vi "Initialize SRQ.vi"(8 "error in":errorcluster {"code" format="%.0x"}, 11 "dup VISA session":refnum<visa-resource-name>) -> (0 "error out (no error)":errorcluster {"code" format="%.0x"}, 3 "dup VISA session":refnum<visa-resource-name>)   [LabVIEW 2011]
doc: "Initializes VISA for a service request, discards any events already in the queue, then enables VISA event handling for a service request.\n\nThis VI is part of an SRQ operation sequence, the order of which is as follows:\n\n1) Set up instrument event-enable registers\n2) Call Initialize SRQ.vi\n3) Perform an operation that causes the instrument to generate a service request\n4) Call Wait on SRQ.vi\n\nor\n\n1) Set up instrument event enable registers\n2) Call Initialize SRQ.vi\n3) Perform the following in parallel using parallel loops or other LV event handling feature:\n - Perform operations that might cause the instrument to generate a service request\n - Call Check on SRQ.vi\n4) Handle any service request received\n5) Call Close SRQ.vi when finished performing instrument operations \n\nUse the following VIs to help you set up the instrument event-enable registers: \n\nSet-Query SRER.vi\nSet-Query SESER.vi\nOther instrument-specific event-enable registers (e.g., Agilent 34401A Questionable Data Event Register)"
uses:
  <vilib>/Instr/_visa.llb/Select Event Type.ctl
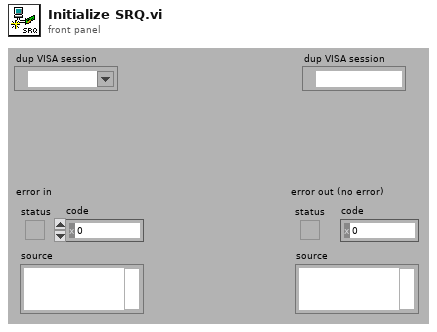
[diagram p1: front panel]
types:
  T1 = typedef "Select Event Type.ctl" = u32
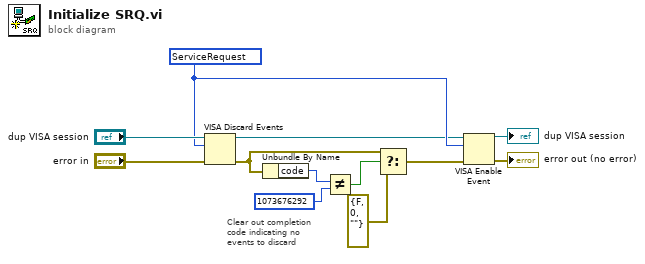
[diagram p0: block diagram]
diagram:
  w10 = T1 1073684491 items=["ServiceRequest"=1073684491, "Trigger"=3221168138, "Clear"=1073684493, "VXI-Signal"=1073684512, "VXI/VME-Interrupt"=3221168161, "VXI/VME-Sysfail"=1073684509, "VXI/VME-Sysreset"=1073684510, "GPIB-CIC"=1073684498, "GPIB-Talk"=1073684499, "GPIB-Listen"=1073684500, "PXI-Interrupt"=1073684514, "AllEnabled"=1073709055] ("Event Type")
  # "Clear out completion\ncode indicating no \nevents to discard"
  n1 = VISA Discard Events(8:"error in", 10:w10, 11:"dup VISA session") -> (0:w5:errorcluster, 3:w9:refnum<visa-resource-name>)  [unwired: 1 in]
  n2 = Unbundle By Name(w5) -> ("code"=w8:i32)
  n3 = Not Equal?(x=w8, y=1073676292 ("code")) -> (x != y?=w6:bool)
  n4 = Select(t=w5, s=w6, f=errorcluster {"status"=FALSE, "code"=0, "source"=""} ("error cluster")) -> (s? t:f=w3:errorcluster)
  n5 = VISA Enable Event(8:w3, 10:w10, 11:w9) -> (0:→"error out (no error)":errorcluster, 3:→"dup VISA session":refnum<visa-resource-name>)  [unwired: 1 in]
